vi "update.get_by_asset.request.vi"(8 "error in":errorcluster, 11 "asset":refnum<class "asset.lvclass">) -> (0 "error out":errorcluster, 1 "Request":string)   [LabVIEW 2020, in "Run.lvclass"]
uses:
  <vilib>/LabVIEW Open Source Project/Epoch Date & Time/epoch.UNIX/Epoch.UNIX.lvclass
  C:/Program Files/National Instruments/LabVIEW 2020/vi.lib/LabVIEW Open Source Project/Epoch Date & Time/epoch/Epoch.lvclass
  <vilib>/LabVIEW Open Source Project/Epoch Date & Time/Get Epoch Time.vi
  Run.lvclass
  Run.lvclass/Run.ctl
  asset/asset.lvclass
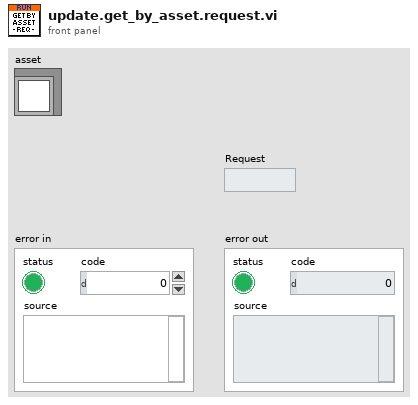
[diagram p1: front panel]
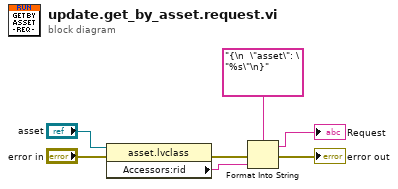
[diagram p0: block diagram]
diagram:
  n1 = property class="asset.lvclass"(reference="asset", error in="error in") -> (error out=w2:errorcluster, "Accessors:rid"=w3:string)  [unwired: 1 out]
  n2 = Format Into String(format string="{\n  \"asset\": \"%s\"\n}", error in=w2, w3) -> (resulting string=→"Request":string, error out=→"error out":errorcluster)  [unwired: 1 in]
